vi "Read Test Method count.vi"(8 "error in (no error)":errorcluster, 11 "Report In":refnum<class "Test Report.lvclass">) -> (0 "error out":errorcluster, 1 "Test Method count string":string, 2 "Test Method count":i32, 3 "Report Out":refnum<class "Test Report.lvclass">)   [LabVIEW 2020, in "Test Report.lvclass"]
uses:
  Test Report.lvclass
  Test Report.lvclass/Test Report.ctl
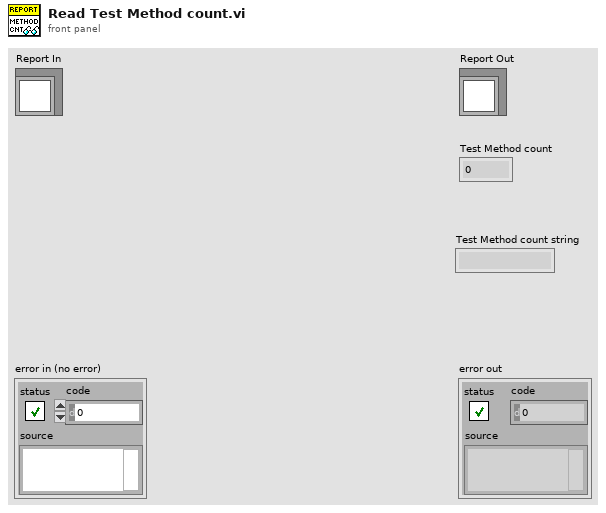
[diagram p1: front panel]
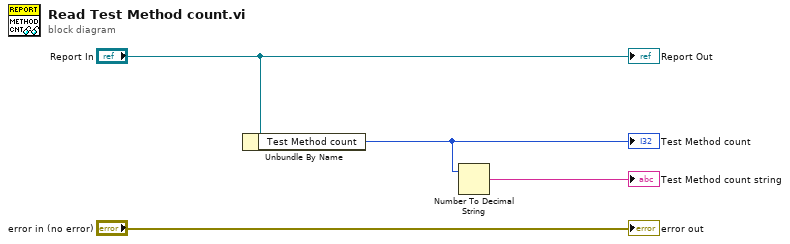
[diagram p0: block diagram]
diagram:
  n1 = Unbundle By Name("Report In") -> ("Test Method count"=w1:i32)
  "Test Method count" <- w1
  n2 = Number To Decimal String(number=w1) -> (decimal integer string=→"Test Method count string":string)  [unwired: 1 in]
  "error out" <- "error in (no error)"
  "Report Out" <- "Report In"
